vi "write tag bus to cvt.vi"(9 "Indices":i32[](array[numeric]), 10 "Data Type":T2, 11 "data table in":T1) -> (3 "data table out":T1)   [LabVIEW 2013, in "TEC runtime.lvclass"]
uses:
  TEC runtime.lvclass
  <vilib>/NI/Current Value Table/Type Defs/Data Types.ctl
  <vilib>/NI/Tag Bus/table/data table.ctl
  <vilib>/NI/Current Value Table/DataTypes/Double_Write Index Set.vi
  <vilib>/NI/Current Value Table/DataTypes/Array of String_Write Index Set.vi
  <vilib>/NI/Current Value Table/DataTypes/Array of Boolean_Write Index Set.vi
  <vilib>/NI/Current Value Table/DataTypes/Array of Single_Write Index Set.vi
  <vilib>/NI/Current Value Table/DataTypes/Array of Double_Write Index Set.vi
  <vilib>/NI/Current Value Table/DataTypes/Array of I8_Write Index Set.vi
  <vilib>/NI/Current Value Table/DataTypes/Array of I16_Write Index Set.vi
  <vilib>/NI/Current Value Table/DataTypes/Array of I32_Write Index Set.vi
  <vilib>/NI/Current Value Table/DataTypes/Array of I64_Write Index Set.vi
  <vilib>/NI/Current Value Table/DataTypes/Array of U64_Write Index Set.vi
  <vilib>/NI/Current Value Table/DataTypes/Array of U32_Write Index Set.vi
  <vilib>/NI/Current Value Table/DataTypes/Array of U16_Write Index Set.vi
  <vilib>/NI/Current Value Table/DataTypes/Array of U8_Write Index Set.vi
  <vilib>/NI/Current Value Table/DataTypes/Boolean_Write Index Set.vi
  <vilib>/NI/Current Value Table/DataTypes/String_Write Index Set.vi
  <vilib>/NI/Current Value Table/DataTypes/U8_Write Index Set.vi
  <vilib>/NI/Current Value Table/DataTypes/U16_Write Index Set.vi
  <vilib>/NI/Current Value Table/DataTypes/U32_Write Index Set.vi
  <vilib>/NI/Current Value Table/DataTypes/U64_Write Index Set.vi
  <vilib>/NI/Current Value Table/DataTypes/I8_Write Index Set.vi
  <vilib>/NI/Current Value Table/DataTypes/I16_Write Index Set.vi
  <vilib>/NI/Current Value Table/DataTypes/I32_Write Index Set.vi
  <vilib>/NI/Current Value Table/DataTypes/I64_Write Index Set.vi
  <vilib>/NI/Current Value Table/DataTypes/Single_Write Index Set.vi
  <vilib>/NI/Current Value Table/Memory Block.vi
  <vilib>/NI/Current Value Table/DataTypes/Double_Memory Block.vi
  <vilib>/NI/Current Value Table/DataTypes/Array of String_Memory Block.vi
  <vilib>/NI/Current Value Table/DataTypes/Array of Boolean_Memory Block.vi
  <vilib>/NI/Current Value Table/DataTypes/Array of Single_Memory Block.vi
  <vilib>/NI/Current Value Table/DataTypes/Array of Double_Memory Block.vi
  <vilib>/NI/Current Value Table/DataTypes/Array of I8_Memory Block.vi
  <vilib>/NI/Current Value Table/DataTypes/Array of I16_Memory Block.vi
  <vilib>/NI/Current Value Table/DataTypes/Array of I32_Memory Block.vi
  <vilib>/NI/Current Value Table/DataTypes/Array of I64_Memory Block.vi
  <vilib>/NI/Current Value Table/DataTypes/Array of U64_Memory Block.vi
  <vilib>/NI/Current Value Table/DataTypes/Array of U32_Memory Block.vi
  <vilib>/NI/Current Value Table/DataTypes/Array of U16_Memory Block.vi
  <vilib>/NI/Current Value Table/DataTypes/Array of U8_Memory Block.vi
  <vilib>/NI/Current Value Table/DataTypes/Boolean_Memory Block.vi
  <vilib>/NI/Current Value Table/DataTypes/String_Memory Block.vi
  <vilib>/NI/Current Value Table/DataTypes/U8_Memory Block.vi
  <vilib>/NI/Current Value Table/DataTypes/U16_Memory Block.vi
  <vilib>/NI/Current Value Table/DataTypes/U32_Memory Block.vi
  <vilib>/NI/Current Value Table/DataTypes/U64_Memory Block.vi
  <vilib>/NI/Current Value Table/DataTypes/I8_Memory Block.vi
  <vilib>/NI/Current Value Table/DataTypes/I16_Memory Block.vi
  <vilib>/NI/Current Value Table/DataTypes/I32_Memory Block.vi
  <vilib>/NI/Current Value Table/DataTypes/I64_Memory Block.vi
  <vilib>/NI/Current Value Table/DataTypes/Single_Memory Block.vi
  <vilib>/NI/Current Value Table/Current Value Table.lvlib
  <vilib>/NI/Tag Bus/table/data table.lvlib
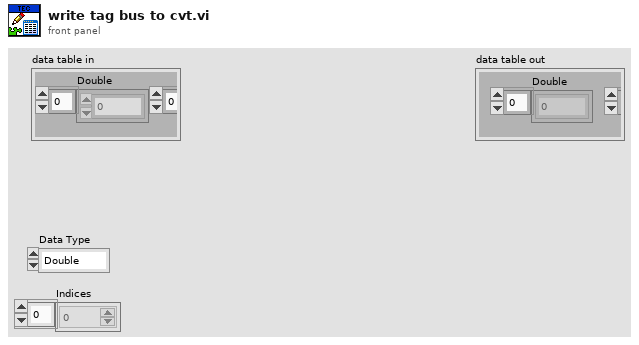
[diagram p1: front panel]
types:
  T1 = typedef "tag bus.lvlib/data table.lvlib/data table.ctl" = cluster{"Double":dbl[], "Single":sgl[], "I64":i64[], "I32":i32[], "I16":i16[], "I8":i8[], "U64":u64[], "U32":u32[], "U16":u16[], "U8":u8[], "Boolean":bool[], "String":string[], "Array of Double":cluster{"DBL Array":dbl[]}[], "Array of Single":cluster{"SGL Array":sgl[]}[], "Array of I64":cluster{"I64 Array":i64[]}[], "Array of I32":cluster{"I32 Array":i32[]}[], "Array of I16":cluster{"I16 Array":i16[]}[], "Array of I8":cluster{"I8 Array":i8[]}[], "Array of U64":cluster{"U64 Array":u64[]}[], "Array of U32":cluster{"U32 Array":u32[]}[], "Array of U16":cluster{"U16 Array":u16[]}[], "Array of U8":cluster{"U8 Array":u8[]}[], "Array of Boolean":cluster{"Boolean Array":bool[]}[], "Array of String":cluster{"String Array":string[]}[]}
  T2 = typedef "Current Value Table.lvlib/Data Types.ctl" = enum16{"Double", "Single", "I64", "I32", "I16", "I8", "U64", "U32", "U16", "U8", "String", "Boolean", "Array of U8", "Array of U16", "Array of U32", "Array of U64", "Array of I64", "Array of I32", "Array of I16", "Array of I8", "Array of Double", "Array of Single", "Array of Boolean", "Array of String"}
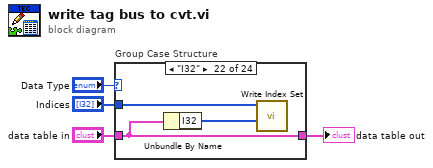
[diagram p0: block diagram]
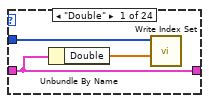
[diagram p2: hidden frame]
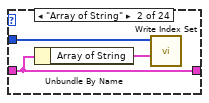
[diagram p3: hidden frame]
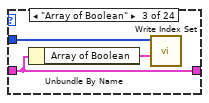
[diagram p4: hidden frame]
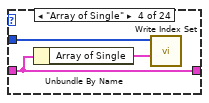
[diagram p5: hidden frame]
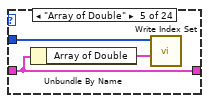
[diagram p6: hidden frame]
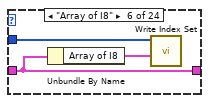
[diagram p7: hidden frame]
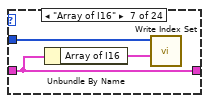
[diagram p8: hidden frame]
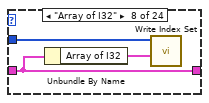
[diagram p9: hidden frame]
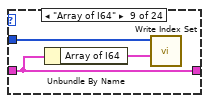
[diagram p10: hidden frame]
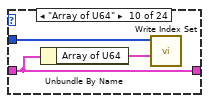
[diagram p11: hidden frame]
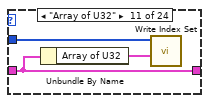
[diagram p12: hidden frame]
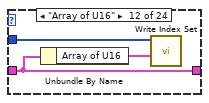
[diagram p13: hidden frame]
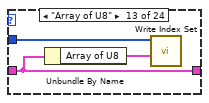
[diagram p14: hidden frame]
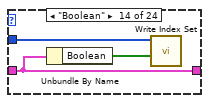
[diagram p15: hidden frame]
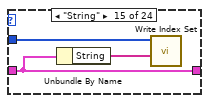
[diagram p16: hidden frame]
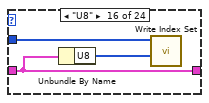
[diagram p17: hidden frame]
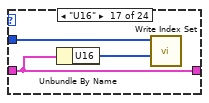
[diagram p18: hidden frame]
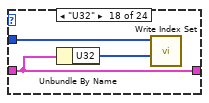
[diagram p19: hidden frame]
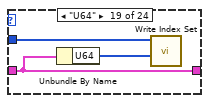
[diagram p20: hidden frame]
diagram:
  n1 = case "Group Case Structure" shown="\"I32\"" "Data Type" {
    tunnel: "data table in" -> [w7 w10 w13 w16 w19 w22 w25 w28 w31 w34 w37 w40 w43 w44 w49 w52 w55 w58 w61 w64 w67 w70 w73 w76]
    tunnel: "Indices" -> [w5 w8 w11 w14 w17 w20 w23 w26 w29 w32 w35 w38 w41 w45 w47 w50 w53 w56 w59 w62 w65 w68 w71 w74]
    tunnel: [w7 w10 w13 w16 w19 w22 w25 w28 w31 w34 w37 w40 w43 w44 w49 w52 w55 w58 w61 w64 w67 w70 w73 w76] -> w2
    frame "Double" {
      n2 = Unbundle By Name(w7) -> ("Double"=w6:dbl[])
      n3 = call-poly <vilib>:"Write Index Set.vi"("Values"=w6, "Indices"=w5) -> ()  [unwired: 10 in]
    }
    frame "Array of String" {
      n4 = Unbundle By Name(w10) -> ("Array of String"=w9:cluster{"String Array":string[]}[])
      n5 = call-poly <vilib>:"Write Index Set.vi"("Values"=w9, "Indices"=w8) -> ()  [unwired: 10 in]
    }
    frame "Array of Boolean" {
      n6 = Unbundle By Name(w13) -> ("Array of Boolean"=w12:cluster{"Boolean Array":bool[]}[])
      n7 = call-poly <vilib>:"Write Index Set.vi"("Values"=w12, "Indices"=w11) -> ()  [unwired: 10 in]
    }
    frame "Array of Single" {
      n8 = Unbundle By Name(w16) -> ("Array of Single"=w15:cluster{"SGL Array":sgl[]}[])
      n9 = call-poly <vilib>:"Write Index Set.vi"("Values"=w15, "Indices"=w14) -> ()  [unwired: 10 in]
    }
    frame "Array of Double" {
      n10 = Unbundle By Name(w19) -> ("Array of Double"=w18:cluster{"DBL Array":dbl[]}[])
      n11 = call-poly <vilib>:"Write Index Set.vi"("Values"=w18, "Indices"=w17) -> ()  [unwired: 10 in]
    }
    frame "Array of I8" {
      n12 = Unbundle By Name(w22) -> ("Array of I8"=w21:cluster{"I8 Array":i8[]}[])
      n13 = call-poly <vilib>:"Write Index Set.vi"("Values"=w21, "Indices"=w20) -> ()  [unwired: 10 in]
    }
    frame "Array of I16" {
      n14 = Unbundle By Name(w25) -> ("Array of I16"=w24:cluster{"I16 Array":i16[]}[])
      n15 = call-poly <vilib>:"Write Index Set.vi"("Values"=w24, "Indices"=w23) -> ()  [unwired: 10 in]
    }
    frame "Array of I32" {
      n16 = Unbundle By Name(w28) -> ("Array of I32"=w27:cluster{"I32 Array":i32[]}[])
      n17 = call-poly <vilib>:"Write Index Set.vi"("Values"=w27, "Indices"=w26) -> ()  [unwired: 10 in]
    }
    frame "Array of I64" {
      n18 = Unbundle By Name(w31) -> ("Array of I64"=w30:cluster{"I64 Array":i64[]}[])
      n19 = call-poly <vilib>:"Write Index Set.vi"("Values"=w30, "Indices"=w29) -> ()  [unwired: 10 in]
    }
    frame "Array of U64" {
      n20 = Unbundle By Name(w34) -> ("Array of U64"=w33:cluster{"U64 Array":u64[]}[])
      n21 = call-poly <vilib>:"Write Index Set.vi"("Values"=w33, "Indices"=w32) -> ()  [unwired: 10 in]
    }
    frame "Array of U32" {
      n22 = Unbundle By Name(w37) -> ("Array of U32"=w36:cluster{"U32 Array":u32[]}[])
      n23 = call-poly <vilib>:"Write Index Set.vi"("Values"=w36, "Indices"=w35) -> ()  [unwired: 10 in]
    }
    frame "Array of U16" {
      n24 = Unbundle By Name(w40) -> ("Array of U16"=w39:cluster{"U16 Array":u16[]}[])
      n25 = call-poly <vilib>:"Write Index Set.vi"("Values"=w39, "Indices"=w38) -> ()  [unwired: 10 in]
    }
    frame "Array of U8" {
      n26 = Unbundle By Name(w43) -> ("Array of U8"=w42:cluster{"U8 Array":u8[]}[])
      n27 = call-poly <vilib>:"Write Index Set.vi"("Values"=w42, "Indices"=w41) -> ()  [unwired: 10 in]
    }
    frame "Boolean" {
      n28 = Unbundle By Name(w44) -> ("Boolean"=w46:bool[])
      n29 = call-poly <vilib>:"Write Index Set.vi"("Values"=w46, "Indices"=w45) -> ()  [unwired: 10 in]
    }
    frame "String" {
      n30 = Unbundle By Name(w49) -> ("String"=w48:string[])
      n31 = call-poly <vilib>:"Write Index Set.vi"("Values"=w48, "Indices"=w47) -> ()  [unwired: 10 in]
    }
    frame "U8" {
      n32 = Unbundle By Name(w52) -> ("U8"=w51:u8[])
      n33 = call-poly <vilib>:"Write Index Set.vi"("Values"=w51, "Indices"=w50) -> ()  [unwired: 10 in]
    }
    frame "U16" {
      n34 = Unbundle By Name(w55) -> ("U16"=w54:u16[])
      n35 = call-poly <vilib>:"Write Index Set.vi"("Values"=w54, "Indices"=w53) -> ()  [unwired: 10 in]
    }
    frame "U32" {
      n36 = Unbundle By Name(w58) -> ("U32"=w57:u32[])
      n37 = call-poly <vilib>:"Write Index Set.vi"("Values"=w57, "Indices"=w56) -> ()  [unwired: 10 in]
    }
    frame "U64" {
      n38 = Unbundle By Name(w61) -> ("U64"=w60:u64[])
      n39 = call-poly <vilib>:"Write Index Set.vi"("Values"=w60, "Indices"=w59) -> ()  [unwired: 10 in]
    }
    frame "I8" {
      n40 = Unbundle By Name(w64) -> ("I8"=w63:i8[])
      n41 = call-poly <vilib>:"Write Index Set.vi"("Values"=w63, "Indices"=w62) -> ()  [unwired: 10 in]
    }
    frame "I16" {
      n42 = Unbundle By Name(w67) -> ("I16"=w66:i16[])
      n43 = call-poly <vilib>:"Write Index Set.vi"("Values"=w66, "Indices"=w65) -> ()  [unwired: 10 in]
    }
    frame "I32" {
      n44 = Unbundle By Name(w70) -> ("I32"=w69:i32[])
      n45 = call-poly <vilib>:"Write Index Set.vi"("Values"=w69, "Indices"=w68) -> ()  [unwired: 10 in]
    }
    frame "I64" {
      n46 = Unbundle By Name(w73) -> ("I64"=w72:i64[])
      n47 = call-poly <vilib>:"Write Index Set.vi"("Values"=w72, "Indices"=w71) -> ()  [unwired: 10 in]
    }
    frame "Single" {
      n48 = Unbundle By Name(w76) -> ("Single"=w75:sgl[])
      n49 = call-poly <vilib>:"Write Index Set.vi"("Values"=w75, "Indices"=w74) -> ()  [unwired: 10 in]
    }
  }
  "data table out" <- w2
